vi "StartFound.vi"(8 "error in (no error)":errorcluster, 10 "String":string, 11 "TCP_Server_Connection_Handler in":refnum<class "TCP_Server_Connection_Handler.lvclass">) -> (0 "error out":errorcluster, 2 "Start?":bool, 3 "TCP_Server_Connection_Handler out":refnum<class "TCP_Server_Connection_Handler.lvclass">)   [LabVIEW 2023, in "TCP_Server_Connection_Handler.lvlib" / "TCP_Server_Connection_Handler.lvclass"]
uses:
  TCP_Server_Connection_Handler.lvclass
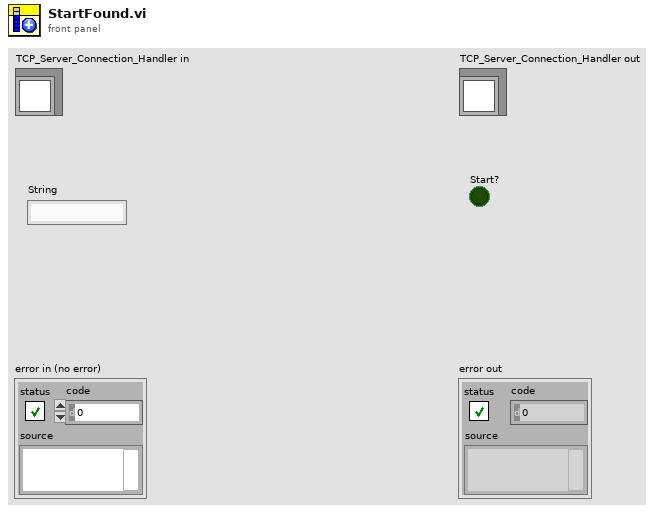
[diagram p1: front panel]
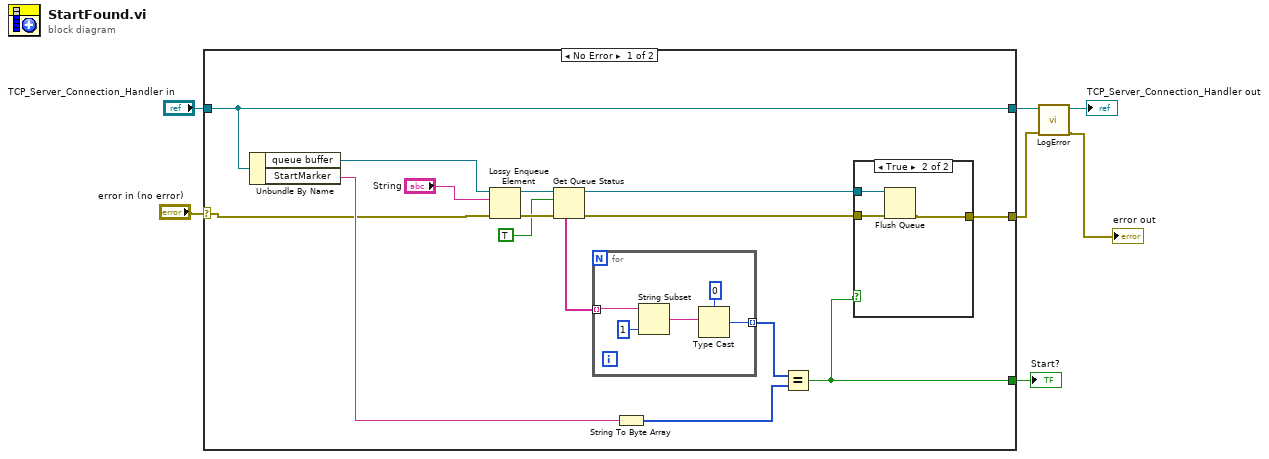
[diagram p0: block diagram]
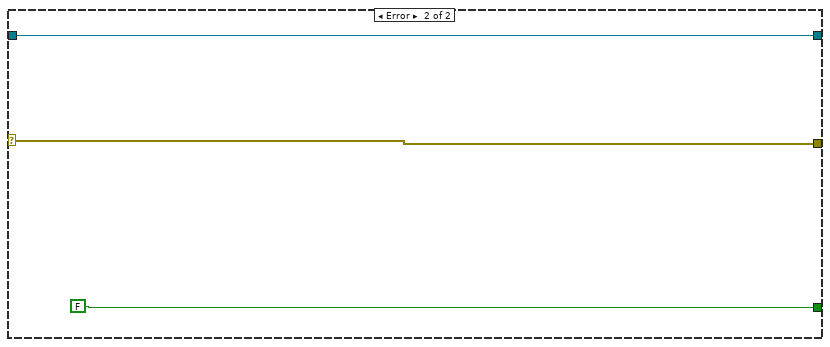
[diagram p3: hidden frame]
diagram:
  n1 = case shown="No Error" "error in (no error)" {
    selector: "error in (no error)" -> [w13 w34]
    tunnel: [w8 w34] -> w2
    tunnel: [w22 w33] -> w4
    tunnel: "TCP_Server_Connection_Handler in" -> [w22 w33]
    tunnel: [w11 FALSE] -> w5
    frame No Error {
      n2 = Unbundle By Name(w22) -> ("queue buffer"=w21:refnum<queue>, "StartMarker"=w14:string)
      n3 = Lossy Enqueue Element(queue=w21, element="String", error in (no error)=w13) -> (queue out=w19:refnum<queue>, error out=w18:errorcluster)  [unwired: 2 out]
      n4 = Get Queue Status(queue=w19, return elements? (F)=TRUE, error in (no error)=w18) -> (queue out=w10:refnum<queue>, error out=w9:errorcluster, elements=w15:string[])  [unwired: 5 out]
      n5 = for {
        tunnel: w15 -> [w31] mode=indexing
        tunnel: [w27] -> w12 mode=indexing
        n6 = String Subset(string=w31, length (rest)=1 ("length (rest)")) -> (substring=w29:string)  [unwired: 1 in]
        n7 = Type Cast(type=u8 0, x=w29) -> (*(type *) &x=w27:u8)
      }
      n8 = String To Byte Array(string=w14) -> (unsigned byte array=w16:u8[])
      n9 = Equal?(x=w12, y=w16) -> (x = y?=w11:bool)
      n10 = case shown="True" w11 {
        tunnel: w10 -> [_ w26]
        tunnel: w9 -> [w23 w25]
        tunnel: [w23 w24] -> w8
        frame False {
        }
        frame True {
          n11 = Flush Queue(queue=w26, error in (no error)=w25) -> (error out=w24:errorcluster)  [unwired: 2 out]
        }
      }
    }
    frame Error {
    }
  }
  "Start?" <- w5
  n12 = call "LogError.vi"("error in (no error)"=w2, "TCP_Server_Connection_Handler in"=w4) -> ("error out"=→"error out":errorcluster, "TCP_Server_Connection_Handler out"=→"TCP_Server_Connection_Handler out":refnum<class "TCP_Server_Connection_Handler.lvclass">)  [unwired: 8 in]
